vi "Detect R Peaks.vi"(0 "Filtered ECG":waveform(dbl)(graph)) -> (1 "R-Wave Locations (s)":dbl[](array[numeric]) format="%.2p", 2 "Coordinates":cluster{dbl[], dbl[]})   [LabVIEW 2018]
uses:
  <vilib>/measure/mamon.llb/Waveform Peak Detection for 1 Chan.vi
  <vilib>/measure/NI_MAPro.lvlib
panel:
  out "Locations + Amplitudes":dbl[][](array[numeric])
  out "Locations":dbl[](array[numeric]) format="%.2p"
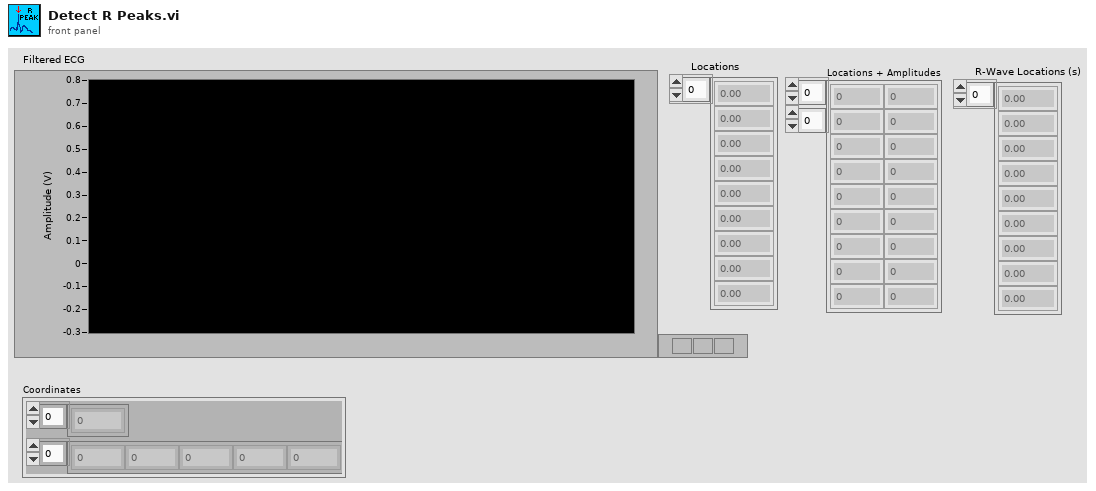
[diagram p1: front panel]
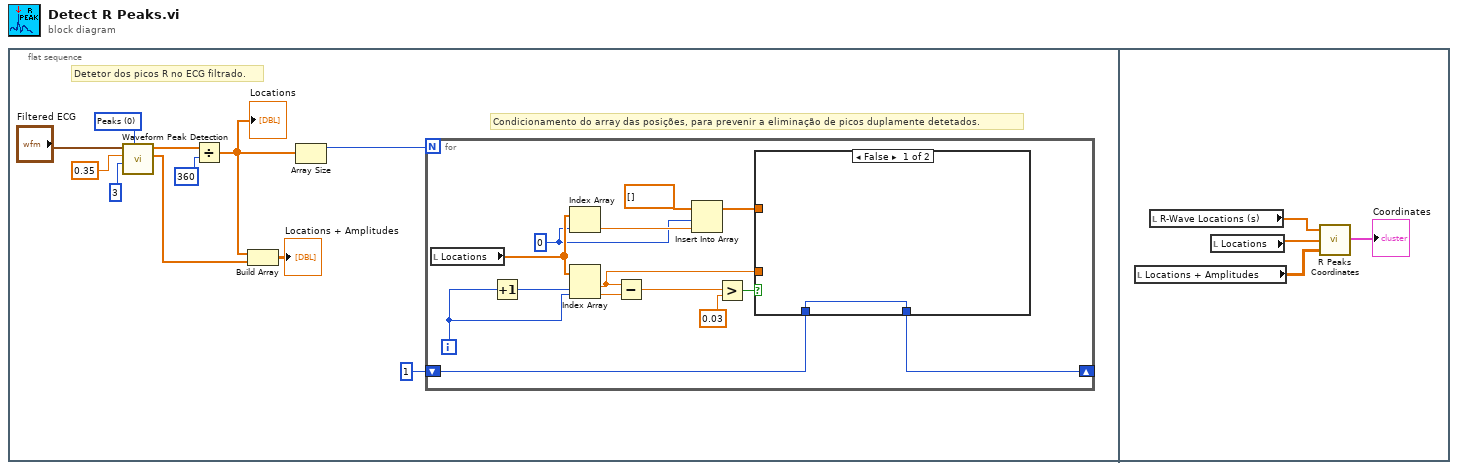
[diagram p0: block diagram]
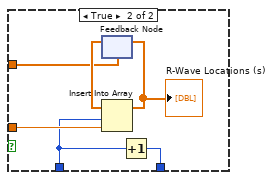
[diagram p2: hidden frame]
diagram:
  n1 = flat-sequence {
    frame #0 {
      w8 = u16 0 items=["Peaks", "Valleys"] ("peaks/valleys")
      # "Condicionamento do array das posições, para prevenir a eliminação de picos duplamente detetados."
      # "Detetor dos picos R no ECG filtrado."
      n2 = call-poly <vilib>:"Waveform Peak Detection.vi"("peaks/valleys"=w8, "width"=3, "threshold"=0.35 ("y"), "Signal In"="Filtered ECG") -> ("Amplitudes"=w2:dbl[], "Locations"=w10:dbl[])  [unwired: 3 in, 3 out]
      n3 = Divide(x=w10, y=360 ("width")) -> (x/y=w3:dbl[])
      "Locations" <- w3
      n4 = Build Array(w3, w2) -> (→"Locations + Amplitudes":dbl[][])
      n5 = Array Size(array=w3) -> (size(s)=w11:i32)
      n6 = for {
        N: w11 -> [_]
        shift-right: [w12] -> _
        shift-left: 1 -> [w13]
        i -> [w14]
        w20 = 0 ("width")
        n7 = local read "Locations"() -> (w22:dbl[])
        n8 = Increment(x=w14) -> (x+1=w15:i32)
        n9 = Index Array(array=w22, index=w20) -> (element=w21:dbl)
        n10 = Index Array(array=w22, index #1=w15, index #2=w14) -> (element #1=w16:dbl, element #2=w17:dbl)
        n11 = Subtract(x=w16, y=w17) -> (x-y=w25:dbl)
        n12 = Insert Into Array(array=dbl[] [], index=w20, new element=w21) -> (w18:dbl[])
        n13 = Greater?(x=w25, y=0.03) -> (0:w23:bool)
        n14 = case shown="False" w23 {
          tunnel: w16 -> [_ w30]
          tunnel: w18 -> [_ w29]
          tunnel: w13 -> [w26 w27]
          tunnel: [w26 w28] -> w12
          frame False {
          }
          frame True {
            n15 = feedback #1(w29) -> (w32:dbl[])
            n16 = Insert Into Array(array=w32, index=w27, new element=w30) -> (w31:dbl[])
            "R-Wave Locations (s)" <- w31
            n17 = feedback-in #1(w31) -> ()
            n18 = Increment(x=w27) -> (x+1=w28:i32)
          }
        }
      }
    }
    frame #1 {
      n19 = local read "Locations + Amplitudes"() -> (w33:dbl[][])
      n20 = local read "R-Wave Locations (s)"() -> (w35:dbl[])
      n21 = local read "Locations"() -> (w34:dbl[])
      n22 = call "R Peaks Coordinates.vi"("2D Loc + Amp"=w33, "Locations"=w34, "R-Wave Location (s)"=w35) -> ("R Peaks Coords"=→"Coordinates":cluster{dbl[], dbl[]})
    }
  }
